vi "log.vi"(6 "接口耗时":i32, 7 "URL":string="URL=", 8 "StartTime":string, 9 "响应报文":string, 10 "header":string, 11 "发送报文":string) -> ()   [LabVIEW 2015]
uses:
  <vilib>/Utility/file.llb/Write Delimited Spreadsheet (string).vi
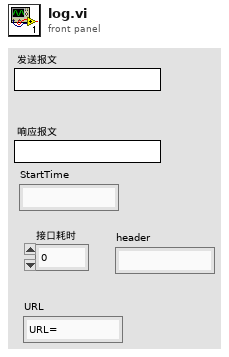
[diagram p1: front panel]
types:
  T1 = enum16{"open", "replace", "create", "open or create", "replace or create", "replace or create with confirmation"}
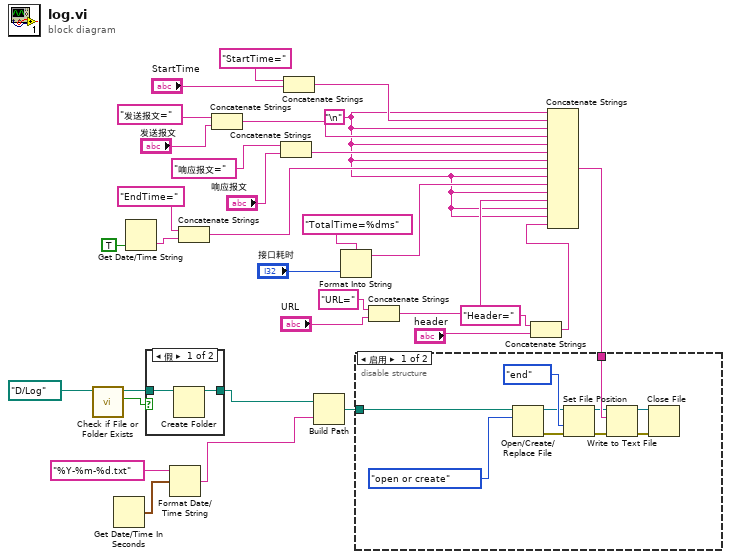
[diagram p0: block diagram]
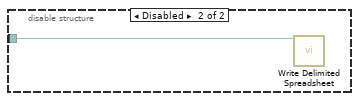
[diagram p2: hidden frame]
diagram:
  w4 = "\n"
  n1 = call <vilib>:"Check if File or Folder Exists.vi"("path"=path "D:/Log" ("路径")) -> ("file or folder exists?"=w28:bool, "dup path"=w29:path)  [unwired: 8 in, 1 out]
  n2 = Get Date/Time In Seconds() -> (seconds since 1Jan1904=w24:timestamp)
  n3 = Get Date/Time String(want seconds? (F)=TRUE ("需要秒？(F)")) -> (time string=w14:string)  [unwired: 2 in, 1 out]
  n4 = case shown="假" w28 {
    tunnel: w29 -> [w34 w35]
    tunnel: [w33 w35] -> w26
    frame False {
      n5 = Create Folder(path (use dialog)=w34) -> (created path=w33:path)  [unwired: 2 in, 2 out]
    }
    frame True {
    }
  }
  n6 = Format Date/Time String(time format string (%c)="%Y-%m-%d.txt" ("时间格式字符串(%c)"), seconds (now)=w24) -> (date/time string=w23:string)  [unwired: 1 in]
  n7 = Concatenate Strings("EndTime=" ("value"), w14) -> (w11:string)
  n8 = Concatenate Strings("发送报文=" ("value"), "发送报文") -> (w17:string)
  n9 = Concatenate Strings("响应报文=" ("value"), "响应报文") -> (w15:string)
  n10 = Concatenate Strings("StartTime=" ("value"), "StartTime") -> (w20:string)
  n11 = Build Path(base path=w26, name or relative path=w23) -> (appended path=w30:path)
  n12 = Format Into String(format string="TotalTime=%dms" ("value"), "接口耗时") -> (resulting string=w8:string)  [unwired: 2 in, 1 out]
  n13 = Concatenate Strings("URL=" ("value"), "URL") -> (w5:string)
  n14 = Concatenate Strings("Header=" ("value"), "header") -> (w1:string)
  n15 = Concatenate Strings(w4, w20, w4, w17, w4, w15, w4, w11, w4, w8, w4, w5, w4, w4, w1) -> (w32:string)
  n16 = disable-structure shown="启用" {
    disable-tunnel: w32 -> [w45 _]
    disable-tunnel: w30 -> [w36 w46]
    frame Enabled {
      n17 = Open/Create/Replace File(file path (use dialog)=w36, operation (0:open)=T1."open or create" ("操作(0:open)")) -> (refnum out=w40:refnum<file>, error out=w41:errorcluster)  [unwired: 4 in, 1 out]
      n18 = Set File Position(refnum=w40, from (0:start)=enum16{"start", "end", "current"}."end" ("自（0:起始）"), error in=w41) -> (refnum out=w42:refnum<file>, error out=w43:errorcluster)  [unwired: 1 in]
      n19 = Write to Text File(file (use dialog)=w42, text=w45, error in=w43) -> (refnum out=w39:refnum<file>, error out=w38:errorcluster)  [unwired: 1 in, 1 out]
      n20 = Close File(refnum=w39, error in=w38) -> ()  [unwired: 2 out]
    }
    frame Disabled {
      n21 = call-poly <vilib>:"Write Delimited Spreadsheet.vi"("file path (dialog if empty)"=w46) -> ()  [unwired: 13 in, 2 out]
    }
  }
